vi "Pre Launch Init.vi"(11 "Nested in":refnum<class "Productos.lvclass">) -> (0 "error out":errorcluster, 3 "Nested out":refnum<class "Productos.lvclass">)   [LabVIEW 2020, in "Productos.lvlib" / "Productos.lvclass"]
doc: "(<B>Filename</B>: Actor Framework.lvlib:Actor.lvclass:Pre Launch Init.vi)\n\nDefines behavior that occurs after the Launch Nested Actor method is invoked but before the actor's Actor Core method begins running.\n\nBy default, this method does nothing. A descendant class may override it to define behavior."
uses:
  Productos.lvclass
  C:/Program Files (x86)/National Instruments/LabVIEW 2020/vi.lib/ActorFramework/Actor/Actor.lvclass
  Productos.lvclass/Productos.ctl
  <vilib>/ActorFramework/Actor/Actor.lvclass/Actor.ctl
  <vilib>/ActorFramework/Message Enqueuer/Message Enqueuer.lvclass/Message Enqueuer.ctl
  <vilib>/ActorFramework/Message Enqueuer/Enqueue.vi
  <vilib>/ActorFramework/Message Enqueuer/Init from Existing Queue.vi
  Productos Messages/Read Inventory Msg/Read Inventory Msg.lvclass
  C:/Program Files (x86)/National Instruments/LabVIEW 2020/vi.lib/ActorFramework/Message/Message.lvclass
  Productos Messages/Initialize Product Msg/Initialize Product Msg.lvclass
  Productos Messages/Open products FP in SP Msg/Open products FP in SP Msg.lvclass
  <vilib>/ActorFramework/Message Priority Queue/Priority Enqueue.vi
  <vilib>/ActorFramework/Message Enqueuer/Message Enqueuer.lvclass
  <vilib>/ActorFramework/Actor/Actor.lvclass
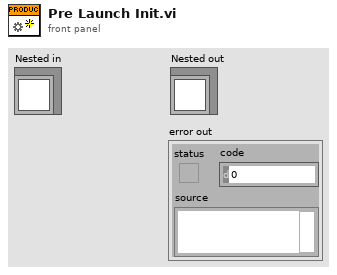
[diagram p1: front panel]
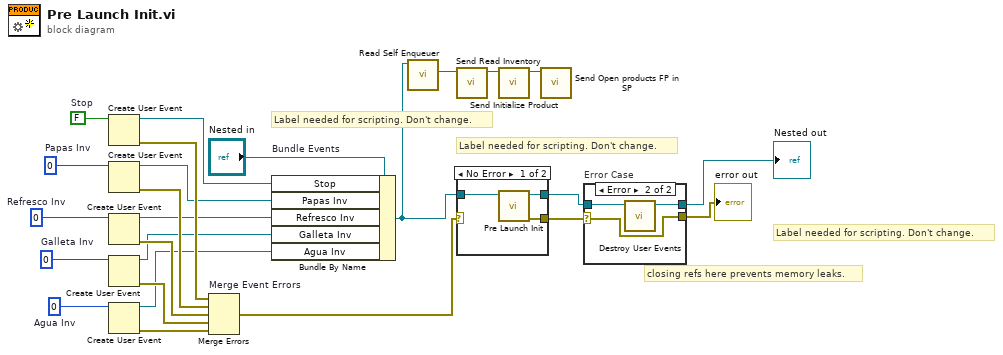
[diagram p0: block diagram]
diagram:
  w3 = 0  # Agua Inv
  w6 = 0  # Galleta Inv
  w9 = 0  # Refresco Inv
  w14 = 0  # Papas Inv
  w24 = FALSE  # Stop
  # "Label needed for scripting. Don't change."
  # "Label needed for scripting. Don't change."
  # "Label needed for scripting. Don't change."
  # "closing refs here prevents memory leaks."
  n1 = Create User Event(user event datatype=w24) -> (user event=w21:refnum<user-event>, error out=w23:errorcluster)  [unwired: 1 in]
  n2 = Create User Event(user event datatype=w14) -> (user event=w13:refnum<user-event>, error out=w12:errorcluster)  [unwired: 1 in]
  n3 = Create User Event(user event datatype=w9) -> (user event=w8:refnum<user-event>, error out=w7:errorcluster)  [unwired: 1 in]
  n4 = Create User Event(user event datatype=w6) -> (user event=w5:refnum<user-event>, error out=w4:errorcluster)  [unwired: 1 in]
  n5 = Create User Event(user event datatype=w3) -> (user event=w2:refnum<user-event>, error out=w1:errorcluster)  [unwired: 1 in]
  n6 = Merge Errors "Merge Event Errors"(w23, w12, w7, w4, w1) -> (w18:errorcluster)
  n7 = Bundle By Name "Bundle Events"(cluster="Nested in", "Stop"=w21, "Papas Inv"=w13, "Refresco Inv"=w8, "Galleta Inv"=w5, "Agua Inv"=w2) -> (w16:refnum<class "Productos.lvclass">)
  n8 = call <vilib>:"Read Self Enqueuer.vi"("Actor"=w16) -> ("Self Enqueuer"=w15:refnum<class "Message Enqueuer.lvclass">)  [unwired: 10 in]
  n9 = call "Send Read Inventory.vi"("Message Enqueuer"=w15) -> ("Message Enqueuer out"=w10:refnum<class "Message Enqueuer.lvclass">)  [unwired: 9 in, 1 out]
  n10 = case shown="No Error" w18 {
    selector: w18 -> [_ w30]
    tunnel: [w28 w29] -> w19
    tunnel: w16 -> [w27 w29]
    tunnel: [w26 w30] -> w17
    frame No Error {
      n11 = call-parent "Pre Launch Init.vi"("Actor in"=w27) -> ("error out"=w26:errorcluster, "Actor out"=w28:refnum<class "Productos.lvclass">)  [unwired: 9 in]
    }
    frame Error {
    }
  }
  n12 = call "Send Initialize Product.vi"("Message Enqueuer"=w10) -> ("Message Enqueuer out"=w11:refnum<class "Message Enqueuer.lvclass">)  [unwired: 9 in, 1 out]
  n13 = call "Send Open products FP in SP.vi"("Message Enqueuer"=w11) -> ()  [unwired: 9 in, 2 out]
  n14 = case "Error Case" shown="Error" w17 {
    selector: w17 -> [w31 w35]
    tunnel: w19 -> [w32 w34]
    tunnel: [w32 w33] -> w22
    tunnel: [w31 w35] -> w20
    frame No Error {
    }
    frame Error {
      n15 = call "Destroy User Events.vi"("UI Template in"=w34) -> ("UI Template out"=w33:refnum<class "Productos.lvclass">)  [unwired: 10 in]
    }
  }
  "error out" <- w20
  "Nested out" <- w22
